vi "Start Call (Exe-Args).vi"(6 "Event References":T3, 7 "Configuration (Default)":T1={"Std Out Stream-Split RegExp Pattern"="\\n", "Std Err Stream-Split RegExp Pattern"="\\n", "ID"="", "Windows UTF8 Conversion"=enum."To OEM Code Page"}, 8 "error in":errorcluster, 9 "Working Directory (default <Not A Path> - System Default)":path=path "" caption="Working Directory", 10 "Arguments (Default: Empty)":string[](array[string]), 11 "Executable Path":path) -> (0 "error out":errorcluster, 3 "New ASE Handle":refnum<class "ase.lvclass">)   [LabVIEW 2020, in "ase.lvlib" / "ase.lvclass"]
doc: "<B>Start an Asynchronous System Executable Call</B>\n\nThe absolute path to the executable should be supplied.\n\nThe User Events References to generate the \"Did Launch\", \"Standard Output\", \"Standard Error\" and \"Did Exit\" events can be supplied or omitted as required. <B>Ensure that the event registration process for any User Events passed to this VI has already been undertaken</B>.\n\nArguments that are to be passed to the executable are specified in an array. Ensure that each argument specifier or value is in a different array element. E.g. to call the ping executable with the arguments \"-n 10 localhost\" use the element values [ -n, 10, localhost]. See the \"examples of the exe-args style calls\" from the boost documentation at https://www.boost.org/doc/libs/1_77_0/doc/html/boost_process/design.html#boost_process.design.arg_cmd_style.\n\n\nThe configuration class allows for override of certain behaviours such as the regular expression used to match the breaks in the Standard Out and Standard Error to be specified.\n\nThis VI generates the following errors:\n-4601: Poorly formatted/incorrect Regular Expression supplied.\n-5691000: Internal Library Error. <Check Error Message for more details>\n-5691301: Unable to launch the executable. <Check Error Message for more details>\n-5691305: Executable paths parameter cannot be an empty value."
uses:
  ase.lvclass
  Event References.ctl
  Standard Output.ctl
  Standard Error.ctl
  Did Exit.ctl
  Configuration.ctl
  Windows UTF8 Conversion Mode.ctl
  ase.lvclass/ase.ctl
  Error Internal Library Implementation Error.vi
  bin/ase_32-3.dll
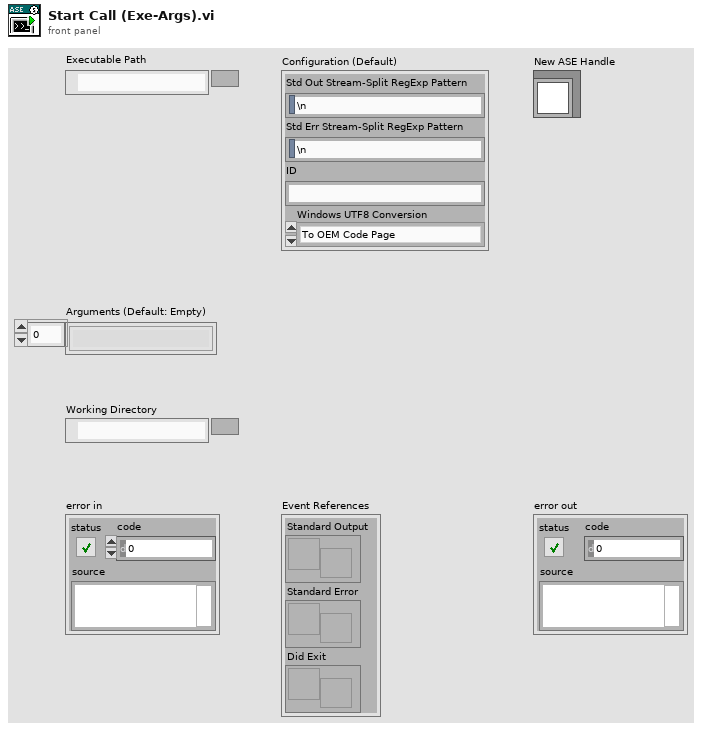
[diagram p1: front panel]
types:
  T1 = typedef "ase.lvlib/ase.lvclass/Configuration.ctl" = cluster{"Std Out Stream-Split RegExp Pattern":string, "Std Err Stream-Split RegExp Pattern":string, "ID":string, "Windows UTF8 Conversion":T2}
  T2 = typedef "ase.lvlib/ase.lvclass/Windows UTF8 Conversion Mode.ctl" = enum8{"None (Pass Through UTF8)", "To ACP Code Page", "To OEM Code Page"}
  T3 = typedef "ase.lvlib/ase.lvclass/Event References.ctl" = cluster{"Standard Output":refnum<user-event>, "Standard Error":refnum<user-event>, "Did Exit":refnum<user-event>}
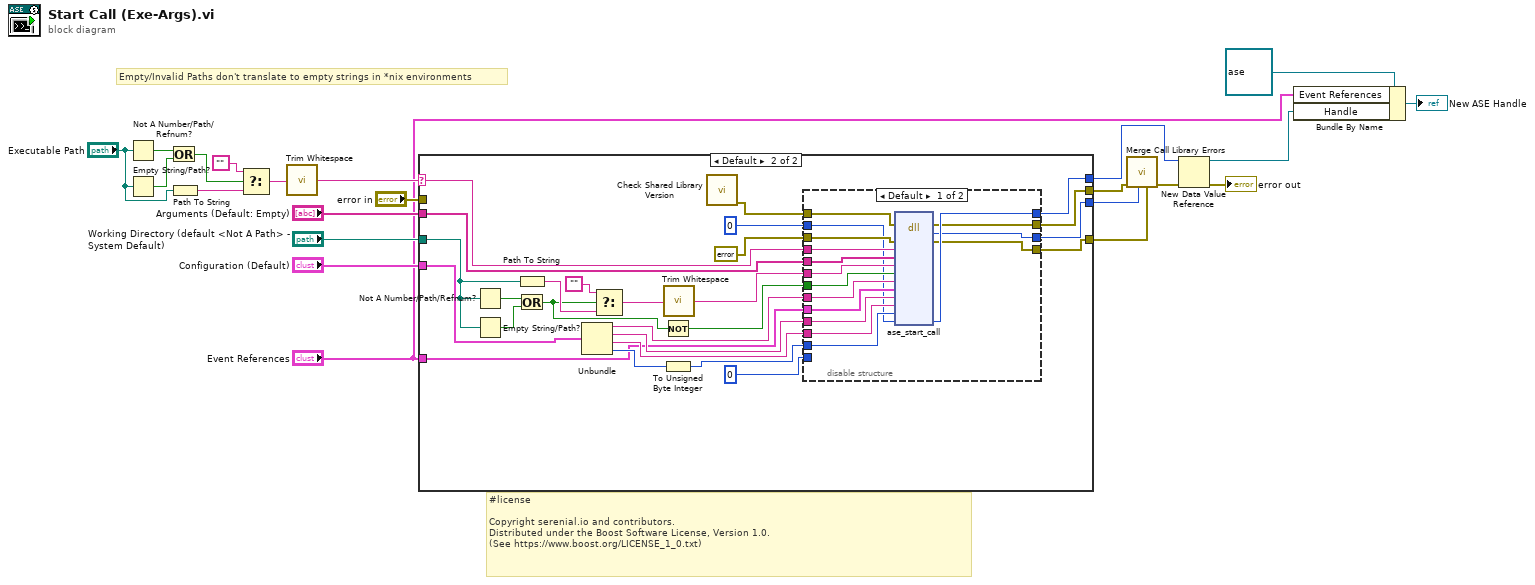
[diagram p0: block diagram]
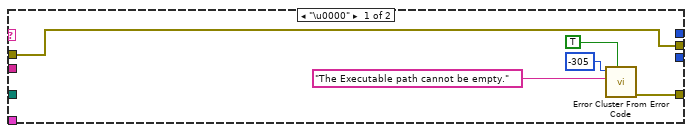
[diagram p2: hidden frame]
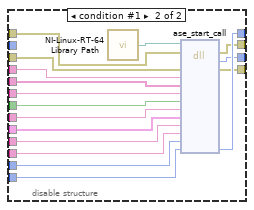
[diagram p3: hidden frame]
diagram:
  # "#license\n\nCopyright serenial.io and contributors.\nDistributed under the Boost Software License, Version 1.0.\n(See https://www.boost.org/LICENSE_1_0.txt)"
  # "Empty/Invalid Paths don't translate to empty strings in *nix environments"
  n1 = Not A Number/Path/Refnum?(number/path/refnum="Executable Path") -> (NaN/Path/Refnum?=w18:bool)
  n2 = Empty String/Path?(string/path="Executable Path") -> (empty?=w19:bool)
  n3 = Or(x=w18, y=w19) -> (x .or. y?=w16:bool)
  n4 = Path To String(path="Executable Path") -> (string=w13:string)
  n5 = Select(t="" ("Empty String Constant"), s=w16, f=w13) -> (s? t:f=w12:string)
  n6 = call "Trim Whitespace.vi"("Input"=w12) -> ("Output"=w4:string)
  n7 = case shown="Default" w4 {
    selector: w4 -> [_ w30]
    tunnel: "Working Directory (default <Not A Path> - System Default)" -> [_ w53]
    tunnel: "Configuration (Default)" -> [_ w52]
    tunnel: [w24 w35] -> w9
    tunnel: [_ w34] -> w8
    tunnel: [w23 w33] -> w7
    tunnel: [_ w32] -> w6
    tunnel: "error in" -> [w24 _]
    tunnel: "Arguments (Default: Empty)" -> [_ w29]
    tunnel: "Event References" -> [_ w28]
    frame "\u0000" {
      n8 = call <vilib>:"Error Cluster From Error Code.vi"("show call chain? (False)"=TRUE, "error message (\"\")"="The Executable path cannot be empty." ("error message (\"\")"), "error code (0)"=-305) -> ("error out"=w23:errorcluster)  [unwired: 6 in]
    }
    frame Default {
      n9 = Not A Number/Path/Refnum?(number/path/refnum=w53) -> (NaN/Path/Refnum?=w46:bool)
      n10 = Empty String/Path?(string/path=w53) -> (empty?=w47:bool)
      n11 = Path To String(path=w53) -> (string=w44:string)
      n12 = Or(x=w46, y=w47) -> (x .or. y?=w41:bool)
      n13 = Unbundle(w52) -> ("Std Out Stream-Split RegExp Pattern"=w39:string, "Std Err Stream-Split RegExp Pattern"=w48:string, "ID"=w38:string, "Windows UTF8 Conversion"=w37:T2)
      n14 = Select(t="" ("Empty String Constant"), s=w41, f=w44) -> (s? t:f=w42:string)
      n15 = Not(x=w41) -> (.not. x?=w40:bool)
      n16 = To Unsigned Byte Integer(number=w37) -> (unsigned 8bit integer=w36:u8)
      n17 = call "Trim Whitespace.vi"("Input"=w42) -> ("Output"=w51:string)
      n18 = call "Check Shared Library Version.vi"() -> ("error out"=w43:errorcluster)  [unwired: 10 in, 1 out]
      n19 = disable-structure "Conditional Disable Structure" shown="Default" {
        disable-tunnel: w43 -> [w67 w85]
        disable-tunnel: errorcluster {"status"=FALSE, "code"=0, "source"=""} ("error in (no error)") -> [w68 w84]
        disable-tunnel: u64 0 ("ASE interface pointer") -> [_ w75]
        disable-tunnel: w48 -> [w61 w78]
        disable-tunnel: w51 -> [w65 w81]
        disable-tunnel: w28 -> [w62 w70]
        disable-tunnel: w30 -> [w69 w83]
        disable-tunnel: w29 -> [w66 w82]
        disable-tunnel: w40 -> [w64 w80]
        disable-tunnel: w39 -> [w63 w79]
        disable-tunnel: w38 -> [w60 w77]
        disable-tunnel: w36 -> [w59 w76]
        disable-tunnel: [w58 w74] -> w32
        disable-tunnel: [w57 w73] -> w35
        disable-tunnel: [w56 w71] -> w34
        disable-tunnel: [w55 w72] -> w33
        disable-tunnel: u64 0 ("handle") -> [w54 _]
        frame condition #0 (active) {
          n20 = dll-call lib="C:/serenial/lib/asynchronous-system-exec/LabVIEW/ase/ase/bin/ase_*-3.*" fn="ase_start_call" ("AsyncSystemExec*.*:wrapperVersion")(error in=w67, "Error Out"=w68, "exe"=w69, "arguments"=w66, "working_directory"=w65, "use_working_directory"=w64, "id"=w63, "event_refs"=w62, "std_out_regex"=w61, "std_err_regex"=w60, "utf8-conversion"=w59, "handle"=w54) -> (error out=w57:errorcluster, "Error Code"=w56:i32, "Error Out"=w55:errorcluster, "handle"=w58:u64)  [unwired: 11 in, 1 out]
        }
        frame condition #1 {
          n21 = call "NI-Linux-RT-64 Library Path.vi"() -> ("Path"=w86:path)
          n22 = dll-call lib="?" fn="ase_start_call" ("AsyncSystemExec*.*:wrapperVersion")(path in=w86, error in=w85, "Error Out"=w84, "exe"=w83, "arguments"=w82, "working_directory"=w81, "use_working_directory"=w80, "id"=w79, "event_refs"=w70, "std_out_regex"=w78, "std_err_regex"=w77, "utf8-conversion"=w76, "handle"=w75) -> (error out=w73:errorcluster, "Error Code"=w71:i32, "Error Out"=w72:errorcluster, "handle"=w74:u64)  [unwired: 10 in, 1 out]
        }
      }
    }
  }
  n23 = call "Merge Call Library Errors.vi"("Library Call Returned Error"=w7, "Error Code"=w8, "error in"=w9) -> ("error IO"=w11:errorcluster)  [unwired: 8 in]
  n24 = New Data Value Reference(data value=w6, error in=w11) -> (data value reference=w5:refnum<data-value>, error out=→"error out":errorcluster)
  n25 = Bundle By Name(cluster=refnum<class "ase.lvclass"> refnum ("serenial.io-ase.lvlib:ase.lvclass"), "Event References"="Event References", "Handle"=w5) -> (→"New ASE Handle":refnum<class "ase.lvclass">)
